vi "Test End.vi"(0 "reference in":refnum<class "Test.lvclass">, 5 "error in (no error)":errorcluster) -> (14 "reference out":refnum<class "Test.lvclass">, 19 "error out":errorcluster)   [LabVIEW 2013, in "Test.lvclass"]
uses:
  Test.lvclass
  Device_class/Device.lvclass
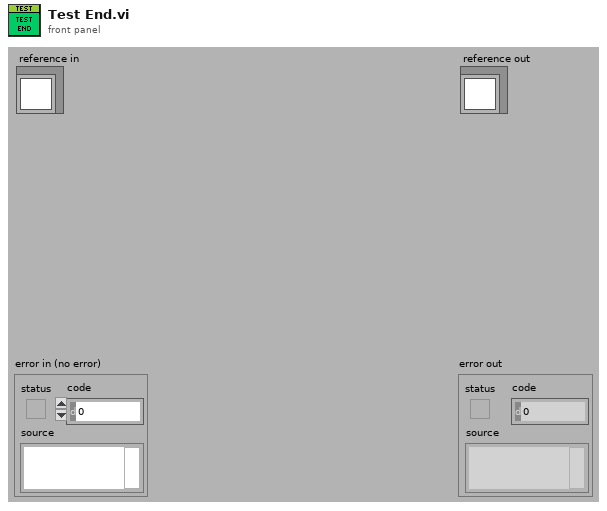
[diagram p1: front panel]
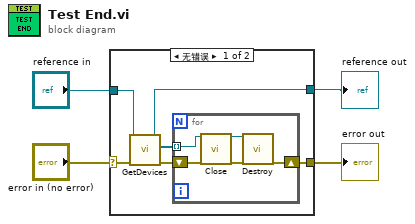
[diagram p0: block diagram]
diagram:
  n1 = case shown="无错误" "error in (no error)" {
    selector: "error in (no error)" -> [w8 w17]
    tunnel: [w5 w17] -> w3
    tunnel: [w9 w16] -> w1
    tunnel: "reference in" -> [w10 w16]
    frame No Error {
      n2 = call-dynamic "GetDevices.vi"("error in (no error)"=w8, "reference in"=w10) -> ("error out"=w7:errorcluster, "Devices"=w6:refnum<class "Device.lvclass">[], "reference out"=w9:refnum<class "Test.lvclass">)  [unwired: 7 in]
      n3 = for {
        shift-right: [w11] -> w5
        shift-left: w7 -> [w15]
        tunnel: w6 -> [w14] mode=indexing
        n4 = call-dynamic "Close.vi"("reference in"=w14, "error in (no error)"=w15) -> ("reference out"=w12:refnum<class "Device.lvclass">, "error out"=w13:errorcluster)  [unwired: 16 in]
        n5 = call-dynamic "Destroy.vi"("reference in"=w12, "error in (no error)"=w13) -> ("error out"=w11:errorcluster)  [unwired: 16 in, 1 out]
      }
    }
    frame Error {
    }
  }
  "error out" <- w3
  "reference out" <- w1
